vi "CalculateBias.vi"(4 "D Coeff":dbl format="%#_13g", 5 "GainV Max V(4.6)":dbl=4.6 format="%#_13g", 6 "GainV tolerence (0.05)":dbl=0.1 format="%#_13g", 7 "Sig target(1.5V)":dbl=1.0 format="%#_13g", 8 "Sig Last(V)":dbl, 9 "GainV Last":dbl=0.1, 10 "Sig Current(V)":dbl, 11 "GainV current":dbl=0.1) -> (3 "V new":dbl)   [LabVIEW 2020]
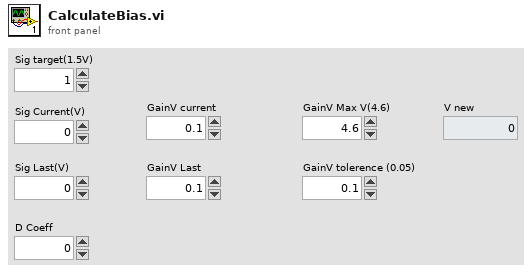
[diagram p1: front panel]
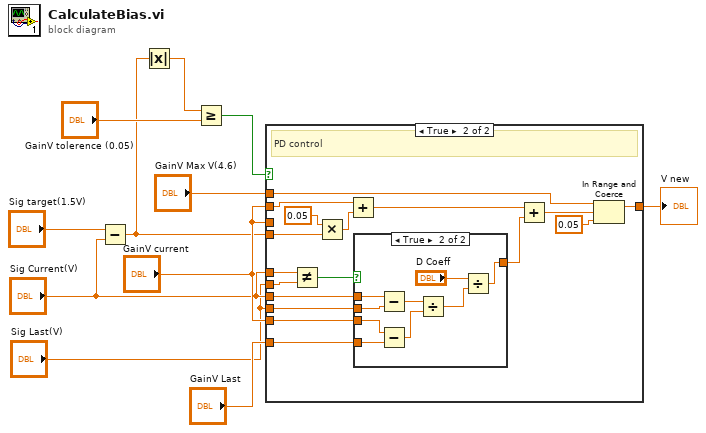
[diagram p0: block diagram]
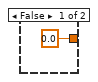
[diagram p3: hidden frame]
diagram:
  n1 = Subtract(x="Sig target(1.5V)", y="Sig Current(V)") -> (x-y=w1:dbl)
  n2 = Absolute Value(x=w1) -> (abs(x)=w9:dbl)
  n3 = Greater Or Equal?(x=w9, y="GainV tolerence (0.05)") -> (x >= y?=w5:bool)
  n4 = case shown="True" w5 {
    tunnel: "GainV current" -> [w12 w26]
    tunnel: [w12 w24] -> w8
    tunnel: w1 -> [_ w27]
    tunnel: "GainV Max V(4.6)" -> [_ w23]
    tunnel: "Sig Current(V)" -> [_ w22]
    tunnel: "Sig Last(V)" -> [_ w21]
    tunnel: "GainV current" -> [_ w20]
    tunnel: "GainV Last" -> [_ w17]
    tunnel: "GainV current" -> [_ _]
    tunnel: "Sig Current(V)" -> [_ w14]
    tunnel: "Sig Last(V)" -> [_ w13]
    frame False {
      # "With in tolerence, no update"
    }
    frame True {
      # "PD control"
      n5 = Not Equal?(x=w14, y=w13) -> (x != y?=w16:bool)
      n6 = Multiply(x=0.05, y=w27) -> (x*y=w29:dbl)
      n7 = Add(x=w26, y=w29) -> (x+y=w19:dbl)
      n8 = case shown="True" w16 {
        tunnel: w22 -> [_ w39]
        tunnel: w21 -> [_ w38]
        tunnel: w20 -> [_ w36]
        tunnel: w17 -> [_ w32]
        tunnel: [0.0 w31] -> w15
        frame False {
        }
        frame True {
          n9 = Subtract(x=w39, y=w38) -> (x-y=w37:dbl)
          n10 = Subtract(x=w36, y=w32) -> (x-y=w35:dbl)
          n11 = Divide(x=w37, y=w35) -> (x/y=w34:dbl)
          n12 = Divide(x="D Coeff", y=w34) -> (x/y=w31:dbl)
        }
      }
      n13 = Add(x=w19, y=w15) -> (x+y=w18:dbl)
      n14 = In Range and Coerce(upper limit=w23, x=w18, lower limit=0.05) -> (coerced(x)=w24:dbl)  [unwired: 1 out]
    }
  }
  "V new" <- w8
